vi "Add Tool From VI.vi"(8 "error in (no error)":errorcluster, 10 "vi path":path, 11 "PyServer in":refnum<class "PyServer.lvclass">) -> (0 "error out":errorcluster, 3 "PyServer out":refnum<class "PyServer.lvclass">)   [LabVIEW 2025, in "Tools.lvlib"]
uses:
  Tools.lvlib
  PyServer/PyServer.lvclass
  PyTool/PyTool.lvclass
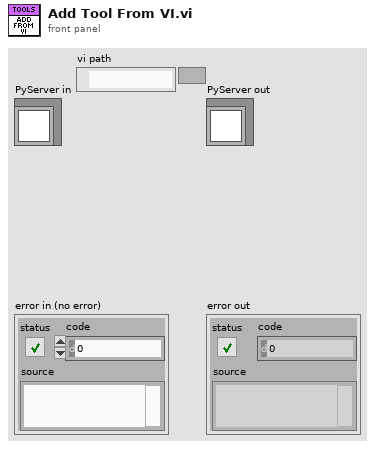
[diagram p1: front panel]
types:
  T1 = typedef "Tools.lvlib/Datatypes.ctl" = enum16{"Float", "Int", "String", "String Array", "Int Array", "Float Array", "Bool Array", "Bool", "Invalid"}
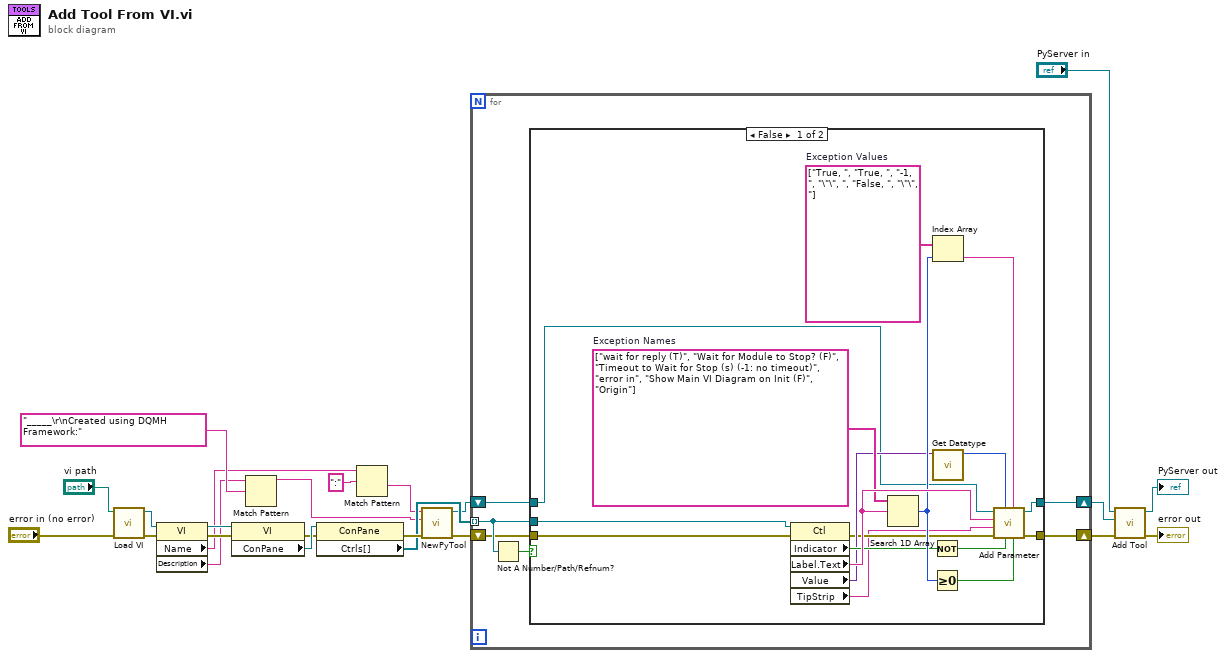
[diagram p0: block diagram]
diagram:
  n1 = call "Load VI.vi"("error in (no error)"="error in (no error)", "vi path"="vi path") -> ("error out"=w10:errorcluster, "VI out"=w9:refnum<vi>)  [unwired: 8 in]
  n2 = property class="VI"(reference=w9, error in=w10) -> (reference out=w19:refnum<vi>, error out=w20:errorcluster, "Name"=w6:string, "Description"=w5:string)
  n3 = property class="VI"(reference=w19, error in=w20) -> (error out=w17:errorcluster, "ConPane"=w18:refnum<vi>)  [unwired: 1 out]
  n4 = Match Pattern(string=w5, regular expression="_____\r\nCreated using DQMH Framework:") -> (before substring=w2:string)  [unwired: 1 in, 3 out]
  n5 = property class="ConPane"(reference=w18, error in=w17) -> (error out=w22:errorcluster, "Ctrls[]"=w21:refnum<vi>[])  [unwired: 1 out]
  n6 = Match Pattern(string=w6, regular expression=":") -> (after substring=w3:string)  [unwired: 1 in, 3 out]
  n7 = call "NewPyTool.vi"("error in (no error)"=w22, "Description"=w2, "Name"=w3) -> ("error out"=w7:errorcluster, "PyTool out"=w4:refnum<class "PyTool.lvclass">)  [unwired: 7 in]
  n8 = for {
    tunnel: w21 -> [w29] mode=indexing
    shift-right: [w25] -> w23
    shift-left: w7 -> [w28]
    shift-right: [w24] -> w1
    shift-left: w4 -> [w26]
    n9 = Not A Number/Path/Refnum?(number/path/refnum=w29) -> (NaN/Path/Refnum?=w27:bool)
    n10 = case shown="False" w27 {
      tunnel: w29 -> [w46 _]
      tunnel: w28 -> [w45 w48]
      tunnel: w26 -> [w32 w47]
      tunnel: [w31 w48] -> w25
      tunnel: [w30 w47] -> w24
      frame False {
        w41 = string[] ["True, ", "True, ", "-1, ", "\"\", ", "False, ", "\"\", "]  # Exception Values
        w43 = string[] ["wait for reply (T)", "Wait for Module to Stop? (F)", "Timeout to Wait for Stop (s) (-1: no timeout)", "error in", "Show Main VI Diagram on Init (F)", "Origin"]  # Exception Names
        n11 = property class="Ctl"(reference=w46, error in=w45) -> (error out=w34:errorcluster, "Indicator"=w40:bool, "Label.Text"=w44:string, "Value"=w39:variant, "TipStrip"=w33:string)  [unwired: 1 out]
        n12 = Search 1D Array(1D array=w43, element=w44) -> (index of element=w42:i32)  [unwired: 1 in]
        n13 = Not(x=w40) -> (.not. x?=w36:bool)
        n14 = Greater Or Equal To 0?(x=w42) -> (x >= 0?=w38:bool)
        n15 = Index Array(array=w41, index=w42) -> (element=w37:string)
        n16 = call "Get Datatype.vi"("Value"=w39) -> ("datatypes"=w35:T1)  [unwired: 10 in]
        n17 = call "Add Parameter.vi"("Ignored?"=w38, "Exception Value"=w37, "Input?"=w36, "type"=w35, "error in (no error)"=w34, "Description"=w33, "Name"=w44, "PyTool in"=w32) -> ("error out"=w31:errorcluster, "PyTool out"=w30:refnum<class "PyTool.lvclass">)  [unwired: 2 in]
      }
      frame True {
      }
    }
  }
  n18 = call "Add Tool.vi"("error in (no error)"=w23, "tool"=w1, "PyServer in"="PyServer in") -> ("error out"=→"error out":errorcluster, "PyServer out"=→"PyServer out":refnum<class "PyServer.lvclass">)  [unwired: 7 in]
